vi "Reader API.vi"(0 "COM":refnum<visa-resource-name>, 1 "Baudrate":u32=19200, 2 "Timeout (ms)":u32=500, 5 "Function":string(combo), 7 "Address":string="X", 11 "error in (no error)":errorcluster, 12 "COM Port Type":T1(ring)=enum."SendWaitRead", 13 "REC":string) -> (4 "ReceiveString":string, 6 "Return":string, 8 "pass?":bool, 15 "error out":errorcluster)   [LabVIEW 2020, in "UART.lvlib"]
uses:
  UART/UART.lvlib
panel:
  in  "Data":string
  # "NOTICE -- YOU MUST LEAVE THIS NOTICE IN PLACE.\n\nCopyright (c) 2017, Fred Guo Guohuijun0422@Gmail.com All rights reserved."
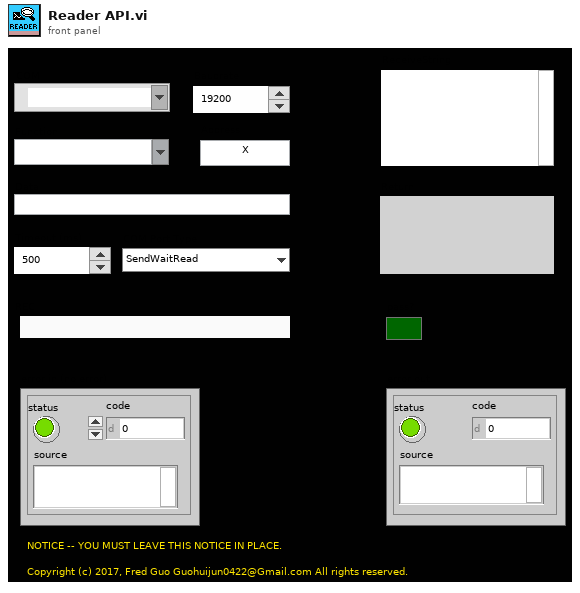
[diagram p1: front panel]
types:
  T1 = enum16{"Open", "Close", "ClearBuffer", "Send", "Read", "SendWaitRead", "SendCompare", "ReadCompare"}
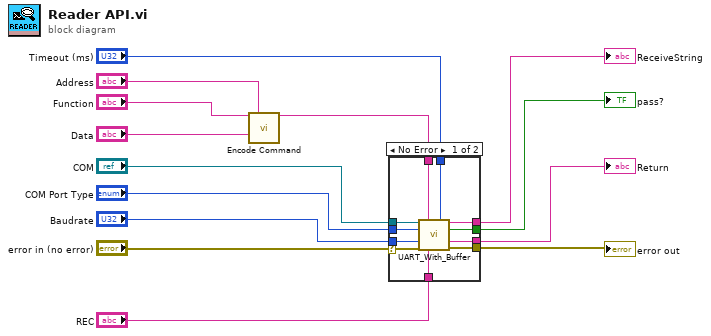
[diagram p0: block diagram]
diagram:
  n1 = call "Encode Command.vi"("Function"="Function", "Address"="Address", "Data"="Data") -> ("Command out"=w14:string)  [unwired: 12 in]
  n2 = case shown="No Error" "error in (no error)" {
    selector: "error in (no error)" -> [w20 w26]
    tunnel: w14 -> [w25 _]
    tunnel: "COM" -> [w24 _]
    tunnel: "Timeout (ms)" -> [w23 _]
    tunnel: "COM Port Type" -> [w22 _]
    tunnel: "Baudrate" -> [w21 _]
    tunnel: "REC" -> [w19 _]
    tunnel: [w18 _] -> w4
    tunnel: [w17 _] -> w3
    tunnel: [w16 _] -> w2
    tunnel: [w15 w26] -> w1
    frame No Error {
      n3 = call "UART_With_Buffer.vi"("COM"=w24, "Send"=w25, "Timeout (ms)"=w23, "Function"=w22, "Baudrate"=w21, "error in (no error)"=w20, "REC"=w19) -> ("ReceiveString"=w18:string, "pass?"=w17:bool, "Return"=w16:string, "error out"=w15:errorcluster)  [unwired: 5 in]
    }
    frame Error {
    }
  }
  "ReceiveString" <- w4
  "pass?" <- w3
  "Return" <- w2
  "error out" <- w1
